vi "Export File - Create Name Value Node.vi"(6 "RootNode in":refnum<k24>, 7 "XmlDocument in":refnum<k24>, 8 "error in (no error)":errorcluster, 9 "Value":string, 10 "Name":string) -> (0 "error out":errorcluster)   [LabVIEW 2019, in "UDP-Custom-Device System Explorer.lvlib"]
uses:
  UDP-Custom-Device System Explorer.lvlib
  System.Xml
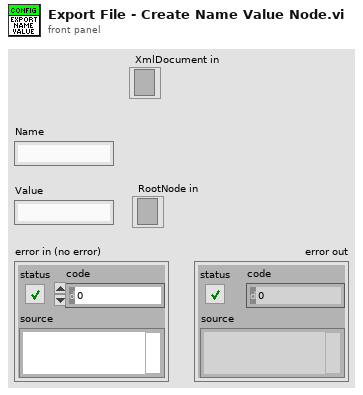
[diagram p1: front panel]
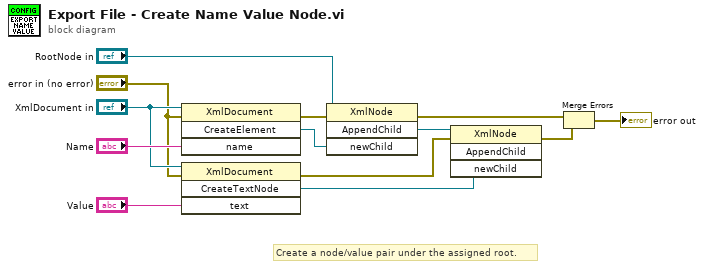
[diagram p0: block diagram]
diagram:
  # "Create a node/value pair under the assigned root."
  n1 = invoke class="XmlDocument" method="CreateElement"(reference="XmlDocument in", error in="error in (no error)", "name"="Name") -> (error out=w11:errorcluster, "CreateElement"=w5:refnum<k24>)  [unwired: 1 in, 2 out]
  n2 = invoke class="XmlDocument" method="CreateTextNode"(reference="XmlDocument in", error in="error in (no error)", "text"="Value") -> (error out=w10:errorcluster, "CreateTextNode"=w12:refnum<k24>)  [unwired: 1 in, 2 out]
  n3 = invoke class="XmlNode" method="AppendChild"(reference="RootNode in", error in=w11, "newChild"=w5) -> (error out=w4:errorcluster, "AppendChild"=w13:refnum<k24>)  [unwired: 1 in, 2 out]
  n4 = invoke class="XmlNode" method="AppendChild"(reference=w13, error in=w10, "newChild"=w12) -> (error out=w3:errorcluster)  [unwired: 1 in, 3 out]
  n5 = Merge Errors(w4, w3) -> (→"error out":errorcluster)
